vi "StickerPrint.vi"(8 "error in":errorcluster caption="错误输入", 11 "Path":string="Config\\2.btw") -> (0 "error out":errorcluster caption="错误输出")   [LabVIEW 2013]
panel:
  out "添加的路径":path
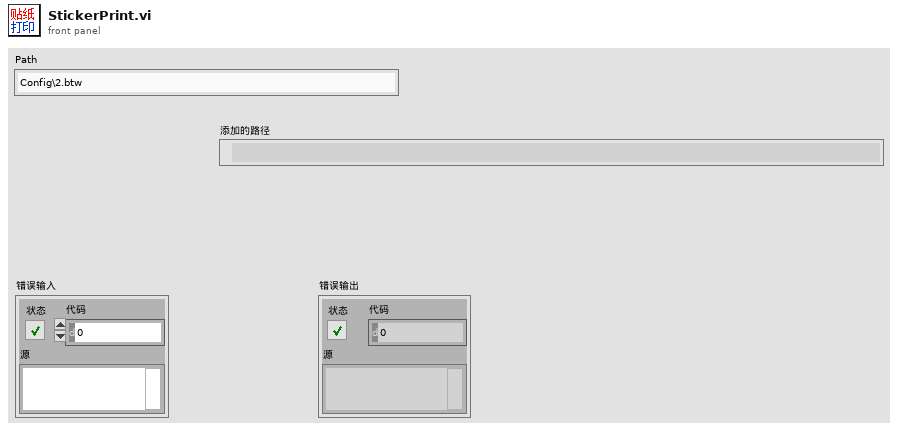
[diagram p1: front panel]
types:
  T1 = enum32{"invalid app kind", "Development System", "Run Time System", "Student Edition", "Embedded LabVIEW", "Evaluation", "Custom"}
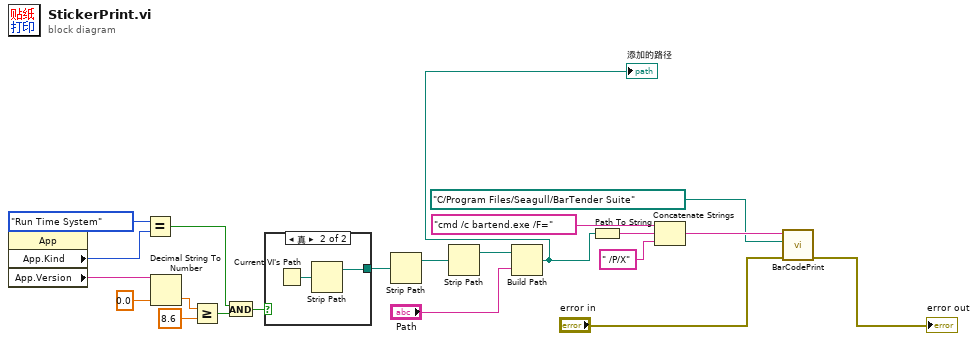
[diagram p0: block diagram]
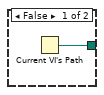
[diagram p2: hidden frame]
diagram:
  n1 = property class="App"() -> ("App.Kind"=w17:T1, "App.Version"=w18:string)  [unwired: 2 in, 2 out]
  n2 = Equal?(x=T1."Run Time System", y=w17) -> (x = y?=w14:bool)
  n3 = Decimal String To Number(string=w18, default (0L)=0.0 ("y")) -> (number=w20:dbl)  [unwired: 1 in, 1 out]
  n4 = Greater Or Equal?(x=w20, y=8.6) -> (x >= y?=w13:bool)
  n5 = And(x=w14, y=w13) -> (x .and. y?=w15:bool)
  n6 = case shown="真" w15 {
    tunnel: [w22 w23] -> w11
    frame False {
      n7 = Current VI's Path() -> (path=w22:path)
    }
    frame True {
      n8 = Current VI's Path() -> (path=w24:path)
      n9 = Strip Path(path=w24) -> (stripped path=w23:path)  [unwired: 1 out]
    }
  }
  n10 = Strip Path(path=w11) -> (stripped path=w10:path)  [unwired: 1 out]
  n11 = Strip Path(path=w10) -> (stripped path=w12:path)  [unwired: 1 out]
  n12 = Build Path(base path=w12, name or relative path="Path") -> (appended path=w7:path)
  "添加的路径" <- w7
  n13 = Path To String(path=w7) -> (string=w6:string)
  n14 = Concatenate Strings("cmd /c bartend.exe /F=" ("命令字符串"), w6, " /P/X") -> (w4:string)
  n15 = call "BarCodePrint.vi"("error in"="error in", "工作目录"=path "C:/Program Files/Seagull/BarTender Suite", "命令字符串"=w4) -> ("error out"=→"error out":errorcluster)  [unwired: 8 in]
